vi "testTTL.vi"() -> ()   [LabVIEW 2015]
panel:
  in  "stop":bool
  out "level":sgl
  out "timestamp (s)":dbl
  out "event on":bool
  in  "channel":u8=1 min=1 max=8
  out "error out":errorcluster
  in  "error in":errorcluster
  in  "port":u16
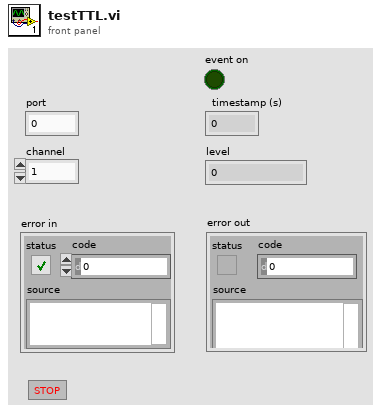
[diagram p1: front panel]
types:
  T1 = enum16{"big-endian, network order", "native, host order", "little-endian"}
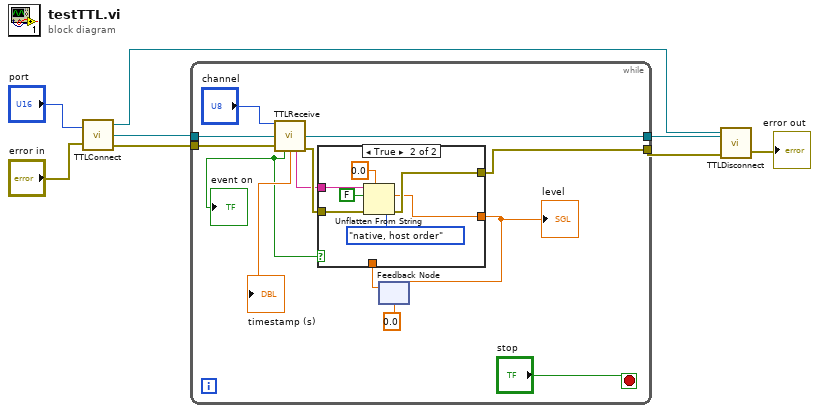
[diagram p0: block diagram]
diagram:
  n1 = call "TTLConnect.vi"("port"="port", "error in"="error in") -> ("context out"=w5:refnum<class "zmq_context.lvclass">, "socket out"=w1:refnum<class "zmq_socket.lvclass">, "error out"=w6:errorcluster)
  n2 = while {
    tunnel: w6 -> [w21]
    tunnel: [w15] -> w4
    tunnel: [w20] -> w2
    tunnel: w1 -> [w19]
    stop <- "stop" stop-if-true
    n3 = call "TTLReceive.vi"("channel"="channel", "socket in"=w19, "error in"=w21) -> ("socket out"=w20:refnum<class "zmq_socket.lvclass">, "event on"=w11:bool, "timestamp (s)"=→"timestamp (s)":dbl, "aux data"=w9:string, "error out"=w16:errorcluster)  [unwired: 7 in, 1 out]
    "event on" <- w11
    n4 = feedback #1(sgl 0.0) -> (w10:sgl)
    n5 = case shown="True" w11 {
      tunnel: w9 -> [_ w30]
      tunnel: w16 -> [w23 w28]
      tunnel: [w23 w27] -> w15
      tunnel: [w22 w26] -> w12
      tunnel: w10 -> [w22 _]
      frame False {
      }
      frame True {
        n6 = Unflatten From String(type=sgl 0.0, binary string=w30, data includes array or string size? (T)=FALSE, byte order (0:big-endian, network order)=T1."native, host order", error in (no error)=w28) -> (value=w26:sgl, error out=w27:errorcluster)  [unwired: 1 out]
      }
    }
    "level" <- w12
    n7 = feedback-in #1(w12) -> ()
  }
  n8 = call "TTLDisconnect.vi"("error in"=w4, "socket in"=w2, "context in"=w5) -> ("error out"=→"error out":errorcluster)  [unwired: 1 in]
